vi "Untitled 3.vi"() -> ()   [LabVIEW 2021]
uses:
  Control 21.ctl
panel:
  in  "Employee 6":T1
  in  "Employee 5":T1
  in  "Employee 4":T1
  in  "Employee 3":T1
  in  "Employee 2":T1
  in  "Employee 1":T1
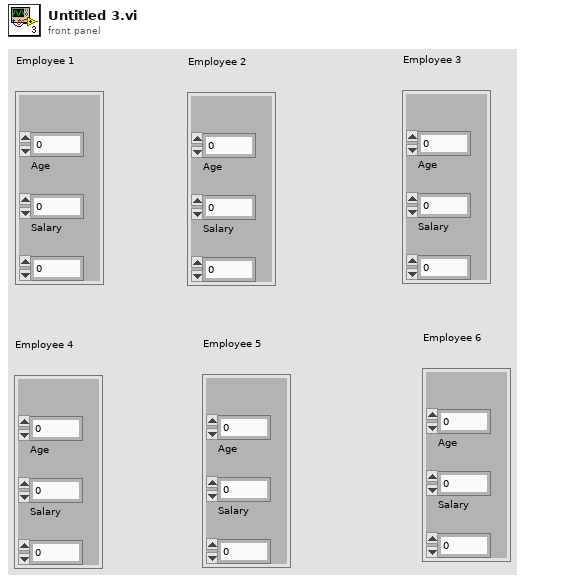
[diagram p1: front panel]
types:
  T1 = typedef "Control 21.ctl" = cluster{"Name":dbl, "Age":dbl, "Salary":dbl}
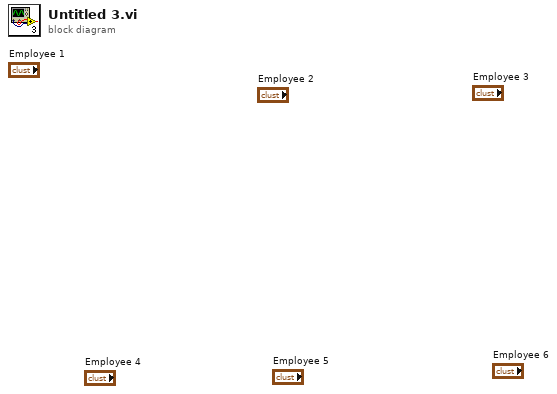
[diagram p0: block diagram]
diagram:
